vi "example_data_simple_pipeline.vi"() -> ()   [LabVIEW 2020]
uses:
  src/vectorstore/vector_qdrant/vector_qdrant.lvclass
  D:/Personal/LabVIEW LLMs/src/vectorstore/abstract_vector_base/abstract_vector_base.lvclass
  src/data_destination/destination_vectorstore/destination_vectorstore.lvclass
  D:/Personal/LabVIEW LLMs/src/data_destination/abstract_datadestination_base/abstract_datadestination_base.lvclass
  src/models/llm_openai_embedding/llm_openai_embedding.lvclass
  D:/Personal/LabVIEW LLMs/src/models/abstract_llm_base/abstract_llm_base.lvclass
  src/data_source/datasource_text_file/datasource_text_file.lvclass
  D:/Personal/LabVIEW LLMs/src/data_source/abstract_datasource_base/abstract_datasource_base.lvclass
  src/data_processor/chunk_character_splitter/chunk_character_splitter.lvclass
  D:/Personal/LabVIEW LLMs/src/data_processor/abstract_dataprocessing_base/abstract_dataprocessing_base.lvclass
  src/data_processor/embed_nodes/embed_nodes.lvclass
  src/models/llm_openai_embedding/Instantiate_llm_openai_embed.vi
  src/data_pipeline/data_simple_pipeline/data_simple_pipeline.lvclass
  src/data_processor/abstract_dataprocessing_base/abstract_dataprocessing_base.lvclass
  src/utilities/env_variables/env_variables.lvlib
panel:
  out "error out":errorcluster
  in  "max_character_length":u32=500
  in  "recursive_folder_load":bool
  in  "model_name":string(combo)="text-embedding-ada-002"
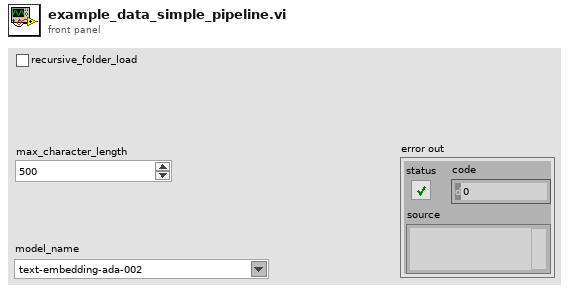
[diagram p1: front panel]
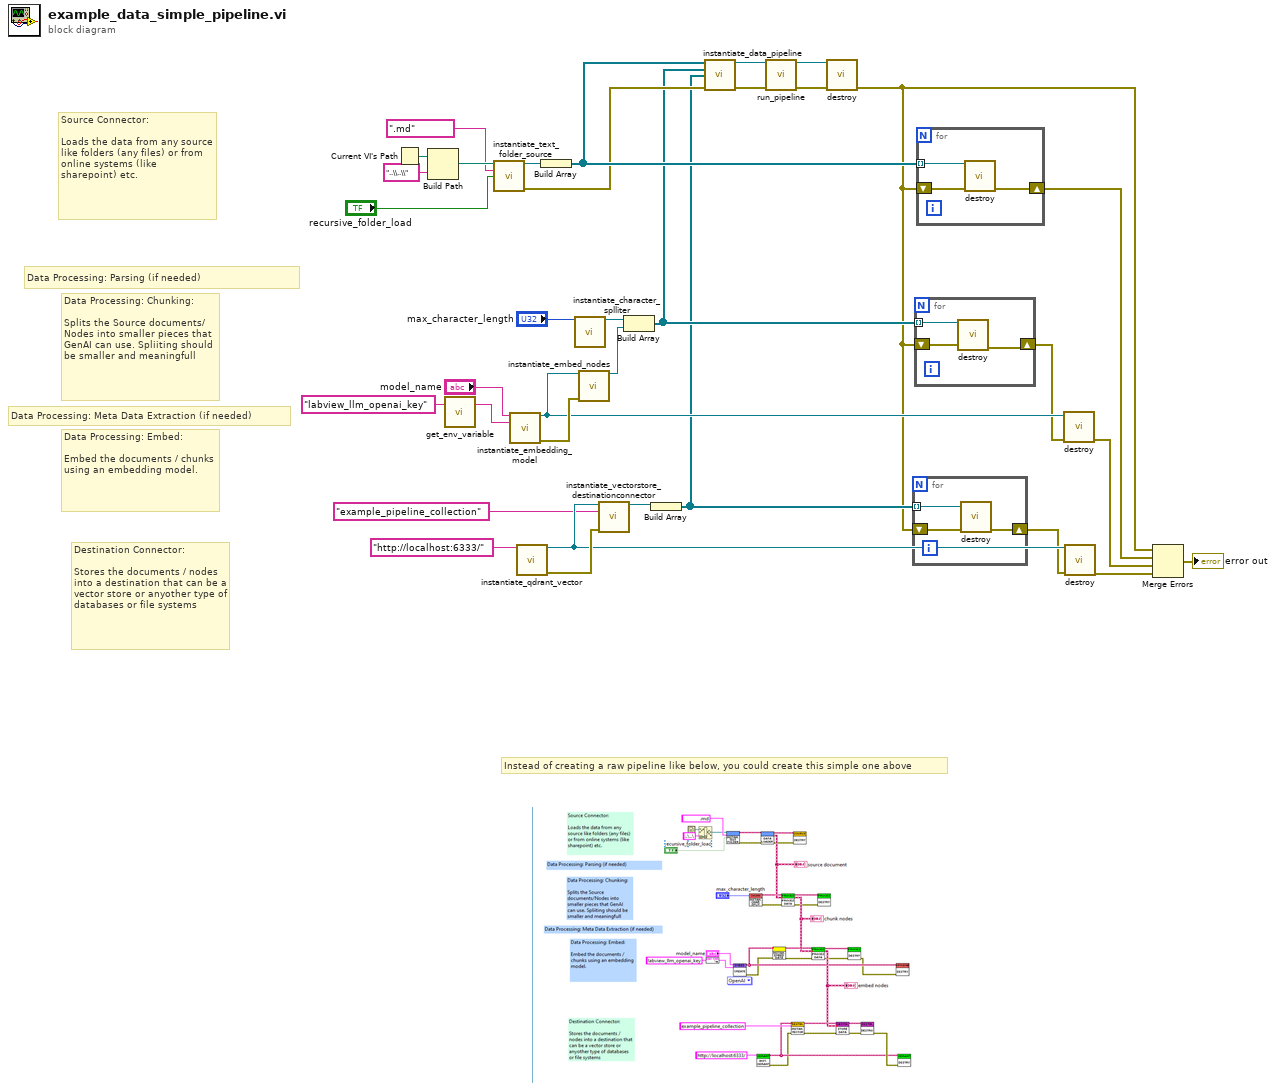
[diagram p0: block diagram]
diagram:
  # "Instead of creating a raw pipeline like below, you could create this simple one above"
  # "Destination Connector:\n\nStores the documents / nodes into a destination that can be a vector store or anyother type of databases or file systems"
  # "Data Processing: Meta Data Extraction (if needed)"
  # "Data Processing: Parsing (if needed)"
  # "Data Processing: Embed:\n\nEmbed the documents / chunks using an embedding model."
  # "Data Processing: Chunking:\n\nSplits the Source documents/Nodes into smaller pieces that GenAI can use. Spliiting should be smaller and meaningfull"
  # "Source Connector:\n\nLoads the data from any source like folders (any files) or from online systems (like sharepoint) etc."
  n1 = Current VI's Path() -> (path=w34:path)
  n2 = Build Path(base path=w34, name or relative path="..\\..\\") -> (appended path=w32:path)
  n3 = call "get_env_variable.vi"("Environment Variable Name"="labview_llm_openai_key") -> ("Value"=w27:string)  [unwired: 1 in, 1 out]
  n4 = call "instantiate_text_folder_source.vi"("source_folder"=w32, "file_extension"=".md", "recursive_folder_load"="recursive_folder_load") -> ("datasource_text_file out"=w14:refnum<class "datasource_text_file.lvclass">, "error out"=w12:errorcluster)  [unwired: 11 in]
  n5 = call-poly "instantiate_embedding_model.vi"("model_name"="model_name", "openai_key"=w27) -> ("llm_openai_embedding out"=w25:refnum<class "llm_openai_embedding.lvclass">, "error out"=w26:errorcluster)  [unwired: 12 in]
  n6 = call "instantiate_qdrant_vector.vi"("host_url"="http://localhost:6333/") -> ("vector_qdrant out"=w22:refnum<class "vector_qdrant.lvclass">, "error out"=w23:errorcluster)  [unwired: 13 in]
  n7 = Build Array(w14) -> (w13:refnum<class "datasource_text_file.lvclass">[])
  n8 = call "instantiate_character_splliter.vi"("max_character_length"="max_character_length") -> ("chunk_character_splitter out"=w11:refnum<class "chunk_character_splitter.lvclass">)  [unwired: 13 in, 1 out]
  n9 = call "instantiate_embed_nodes.vi"("abstract_llm_embedding"=w25, "error in (no error)"=w26) -> ("embed_nodes out"=w10:refnum<class "embed_nodes.lvclass">)  [unwired: 12 in, 1 out]
  n10 = call "instantiate_vectorstore_destinationconnector.vi"("abstract_vector_base"=w22, "store_id"="example_pipeline_collection", "error in (no error)"=w23) -> ("destination_vectorstore out"=w7:refnum<class "destination_vectorstore.lvclass">)  [unwired: 11 in, 1 out]
  n11 = Build Array(w11, w10) -> (w9:refnum<class "abstract_dataprocessing_base.lvclass">[])
  n12 = Build Array(w7) -> (w6:refnum<class "destination_vectorstore.lvclass">[])
  n13 = call "instantiate_data_pipeline.vi"("sources"=w13, "processing steps"=w9, "destinations"=w6, "error in (no error)"=w12) -> ("data_simple_pipeline out"=w18:refnum<class "data_simple_pipeline.lvclass">, "error out"=w17:errorcluster)  [unwired: 10 in]
  n14 = call-dynamic "run_pipeline.vi"("data_simple_pipeline in"=w18, "error in (no error)"=w17) -> ("data_simple_pipeline out"=w16:refnum<class "data_simple_pipeline.lvclass">, "error out"=w15:errorcluster)  [unwired: 12 in]
  n15 = call-dynamic "destroy.vi"("data_simple_pipeline in"=w16, "error in (no error)"=w15) -> ("error out"=w2:errorcluster)  [unwired: 12 in, 1 out]
  n16 = for {
    shift-right: [w37] -> w21
    shift-left: w2 -> [w36]
    tunnel: w6 -> [w35] mode=indexing
    n17 = call-dynamic "destroy.vi"("abstract_datadestination_base in"=w35, "error in (no error)"=w36) -> ("error out"=w37:errorcluster)  [unwired: 12 in, 1 out]
  }
  n18 = for {
    tunnel: w9 -> [w40] mode=indexing
    shift-right: [w38] -> w8
    shift-left: w2 -> [w39]
    n19 = call-dynamic "destroy.vi"("abstract_dataprocessing_base in"=w40, "error in (no error)"=w39) -> ("error out"=w38:errorcluster)  [unwired: 12 in, 1 out]
  }
  n20 = for {
    tunnel: w13 -> [w43] mode=indexing
    shift-right: [w41] -> w3
    shift-left: w2 -> [w42]
    n21 = call-dynamic "destroy.vi"("abstract_datasource_base in"=w43, "error in (no error)"=w42) -> ("error out"=w41:errorcluster)  [unwired: 12 in, 1 out]
  }
  n22 = call-dynamic "destroy.vi"("error in (no error)"=w8, "llm_openai_embedding in"=w25) -> ("error out"=w4:errorcluster)  [unwired: 8 in, 1 out]
  n23 = call-dynamic "destroy.vi"("vector_qdrant in"=w22, "error in (no error)"=w21) -> ("error out"=w5:errorcluster)  [unwired: 12 in, 1 out]
  n24 = Merge Errors(w2, w3, w4, w5) -> (→"error out":errorcluster)
